vi "test_F9P.vi"() -> ()   [LabVIEW 2019] (continued)
4,3,13,13,50,315,39,14,76,037,34,28,59,310,,33,72,237,,3*7B\r\n$GBGSV,4,4,13,34,13,141,,3*47\r\n$GNGLL,3723.61643,N,12656.96813,E,064251.00,A,A*73\r\n$GNRMC,064252.00,A,3723.61654,N,12656.96823,E,0.024,,250720,,,A,V*12\r\n$GNVTG,,T,,M,0.024,N,0.044,K,A*3B\r\n$GNGGA,064252.00,3723.61654,N,12656.96823,E,1,12,0.61,43.2,M,18.5,M,,*7D\r\n$GNGSA,A,3,17,19,06,05,02,12,09,,,,,,1.08,0.61,0.89,1*0B\r\n$GNGSA,A,3,85,70,71,72,,,,,,,,,1.08,0.61,0.89,2*04\r\n$GNGSA,A,3,36,19,11,04,09,12,,,,,,,1.08,0.61,0.89,3*0F\r\n$GNGSA,A,3,28,14,13,11,33,08,10,,,,,,1.08,0.61,0.89,4*0F\r\n$GPGSV,4,1,13,02,65,334,43,04,08,037,40,05,48,261,36,06,58,076,43,1*69\r\n$GPGSV,4,2,13,07,06,105,23,09,38,057,45,12,18,263,31,13,08,191,24,1*6F\r\n$GPGSV,4,3,13,17,19,158,23,19,37,161,34,25,11,294,25,29,07,323,17,1*68\r\n$GPGSV,4,4,13,30,01,134,,1*52\r\n$GPGSV,4,1,13,02,65,334,,04,08,037,26,05,48,261,31,06,58,076,37,6*6D\r\n$GPGSV,4,2,13,07,06,105,,09,38,057,36,12,18,263,17,13,08,191,,6*6F\r\n$GPGSV,4,3,13,17,19,158,26,19,37,161,,25,11,294,,29,07,323,,6*6C\r\n$GPGSV,4,4,13,30,01,134,,6*55\r\n$GLGSV,2,1,06,70,55,030,38,71,68,223,26,72,17,216,42,84,09,133,09,1*70\r\n$GLGSV,2,2,06,85,63,111,27,86,51,337,,1*7F\r\n$GLGSV,2,1,06,70,55,030,,71,68,223,19,72,17,216,26,84,09,133,15,3*7A\r\n$GLGSV,2,2,06,85,63,111,28,86,51,337,21,3*71\r\n$GAGSV,3,1,09,02,04,287,12,04,68,085,37,09,44,196,23,11,78,037,39,7*74\r\n$GAGSV,3,2,09,12,32,115,35,18,55,284,40,19,17,042,31,25,01,241,,7*72\r\n$GAGSV,3,3,09,36,35,314,27,7*4A\r\n$GAGSV,3,1,09,02,04,287,,04,68,085,32,09,44,196,23,11,78,037,30,2*7E\r\n$GAGSV,3,2,09,12,32,115,26,18,55,284,35,19,17,042,27,25,01,241,,2*70\r\n$GAGSV,3,3,09,36,35,314,28,2*40\r\n$GBGSV,4,1,13,04,35,133,,05,09,257,,06,27,182,,07,09,201,18,1*72\r\n$GBGSV,4,2,13,08,65,355,41,09,07,194,,10,16,222,27,11,37,142,33,1*7F\r\n$GBGSV,4,3,13,13,50,315,35,14,76,037,41,28,59,310,36,33,72,237,29,1*79\r\n$GBGSV,4,4,13,34,13,141,,1*45\r\n$GBGSV,4,1,13,04,35,133,,05,09,257,,06,27,182,,07,09,201,,3*79\r\n$GBGSV,4,2,13,08,65,355,36,09,07,194,,10,16,222,18,11,37,142,32,3*70\r\n$GBGSV,4,3,13,13,50,315,39,14,76,037,33,28,59,310,,33,72,237,,3*7C\r\n$GBGSV,4,4,13,34,13,141,,3*47\r\n$GNGLL,3723.61654,N,12656.96823,E,064252.00,A,A*75\r\n$GNRMC,064253.00,A,3723.61656,N,12656.96832,E,0.099,,250720,,,A,V*17\r\n$GNVTG,,T,,M,0.099,N,0.183,K,A*37\r\n$GNGGA,064253.00,3723.61656,N,12656.96832,E,1,12,0.62,43.3,M,18.5,M,,*7C\r\n$GNGSA,A,3,17,19,06,05,02,12,09,,,,,,1.08,0.62,0.88,1*09\r\n$GNGSA,A,3,85,70,71,72,,,,,,,,,1.08,0.62,0.88,2*06\r\n$GNGSA,A,3,36,19,11,04,09,12,,,,,,,1.08,0.62,0.88,3*0D\r\n$GNGSA,A,3,28,14,13,11,33,08,10,,,,,,1.08,0.62,0.88,4*0D\r\n$GPGSV,4,1,13,02,65,334,43,04,08,037,36,05,48,261,36,06,58,076,45,1*6E\r\n$GPGSV,4,2,13,07,06,105,,09,38,057,44,12,18,263,23,13,08,191,25,1*6D\r\n$GPGSV,4,3,13,17,19,158,23,19,37,161,29,25,11,294,24,29,07,323,17,1*65\r\n$GPGSV,4,4,13,30,01,134,,1*52\r\n$GPGSV,4,1,13,02,65,334,,04,08,037,24,05,48,261,31,06,58,076,36,6*6E\r\n$GPGSV,4,2,13,07,06,105,,09,38,057,36,12,18,263,17,13,08,191,,6*6F\r\n$GPGSV,4,3,13,17,19,158,26,19,37,161,,25,11,294,,29,07,323,,6*6C\r\n$GPGSV,4,4,13,30,01,134,,6*55\r\n$GLGSV,2,1,06,70,55,030,38,71,68,223,25,72,17,216,37,84,09,133,13,1*7A\r\n$GLGSV,2,2,06,85,63,111,27,86,51,337,,1*7F\r\n$GLGSV,2,1,06,70,55,030,,71,68,223,19,72,17,216,26,84,09,133,12,3*7D\r\n$GLGSV,2,2,06,85,63,111,30,86,51,337,17,3*7D\r\n$GAGSV,3,1,09,02,04,287,09,04,68,085,39,09,44,196,30,11,78,037,38,7*73\r\n$GAGSV,3,2,09,12,32,115,30,18,55,284,33,19,17,042,31,25,01,241,,7*73\r\n$GAGSV,3,3,09,36,35,314,32,7*4E\r\n$GAGSV,3,1,09,02,04,287,,04,68,085,33,09,44,196,23,11,78,037,31,2*7E\r\n$GAGSV,3,2,09,12,32,115,26,18,55,284,35,19,17,042,26,25,01,241,,2*71\r\n$GAGSV,3,3,09,36,35,314,28,2*40\r\n$GBGSV,4,1,13,04,35,133,,05,09,257,,06,27,182,,07,09,201,20,1*79\r\n$GBGSV,4,2,13,08,65,355,39,09,07,194,,10,16,222,24,11,37,142,27,1*76\r\n$GBGSV,4,3,13,13,50,315,35,14,76,037,41,28,59,310,39,33,73,239,28,1*78\r\n$GBGSV,4,4,13,34,13,141,,1*45\r\n$GBGSV,4,1,13,04,35,133,,05,09,257,,06,27,182,,07,09,201,,3*79\r\n$GBGSV,4,2,13,08,65,355,37,09,07,194,,10,16,222,17,11,37,142,25,3*78\r\n$GBGSV,4,3,13,13,50,315,39,14,76,037,34,28,59,310,,33,73,239,,3*74\r\n$GBGSV,4,4,13,34,13,141,,3*47\r\n$GNGLL,3723.61656,N,12656.96832,E,064253.00,A,A*76\r\n$GNRMC,064254.00,A,3723.61658,N,12656.96838,E,0.064,,250720,,,A,V*16\r\n$GNVTG,,T,,M,0.064,N,0.118,K,A*37\r\n$GNGGA,064254.00,3723.61658,N,12656.96838,E,1,12,0.63,43.3,M,18.5,M,,*7E\r\n$GNGSA,A,3,17,19,06,05,02,12,09,,,,,,1.11,0.63,0.91,1*08\r\n$GNGSA,A,3,85,70,71,72,,,,,,,,,1.11,0.63,0.91,2*07\r\n$GNGSA,A,3,36,19,11,04,09,12,,,,,,,1.11,0.63,0.91,3*0C\r\n$GNGSA,A,3,28,14,13,11,33,08,10,,,,,,1.11,0.63,0.91,4*0C\r\n$GPGSV,4,1,13,02,65,334,46,04,08,037,36,05,48,261,36,06,58,076,44,1*6A\r\n$GPGSV,4,2,13,07,06,105,,09,38,057,48,12,18,263,25,13,08,191,22,1*60\r\n$GPGSV,4,3,13,17,19,158,24,19,37,161,33,25,11,294,22,29,07,323,21,1*6A\r\n$GPGSV,4,4,13,30,01,134,,1*52\r\n$GPGSV,4,1,13,02,65,334,,04,08,037,25,05,48,261,30,06,58,076,20,6*69\r\n$GPGSV,4,2,13,07,06,105,,09,38,057,38,12,18,263,16,13,08,191,,6*60\r\n$GPGSV,4,3,13,17,19,158,22,19,37,161,,25,11,294,,29,07,323,,6*68\r\n$GPGSV,4,4,13,30,01,134,,6*55\r\n$GLGSV,2,1,06,70,55,030,38,71,68,223,25,72,17,216,42,84,09,133,11,1*7A\r\n$GLGSV,2,2,06,85,63,111,34,86,51,337,,1*7D\r\n$GLGSV,2,1,06,70,55,030,,71,68,223,16,72,17,216,24,84,09,133,15,3*77\r\n$GLGSV,2,2,06,85,63,111,21,86,51,337,13,3*79\r\n$GAGSV,3,1,09,02,04,287,09,04,68,085,39,09,44,196,31,11,78,037,38,7*72\r\n$GAGSV,3,2,09,12,32,115,27,18,55,284,31,19,17,042,34,25,01,241,,7*72\r\n$GAGSV,3,3,09,36,35,314,28,7*45\r\n$GAGSV,3,1,09,02,04,287,,04,68,085,35,09,44,196,25,11,78,037,32,2*7D\r\n$GAGSV,3,2,09,12,32,115,29,18,55,284,36,19,17,042,32,25,01,241,,2*78\r\n$GAGSV,3,3,09,36,35,314,28,2*40\r\n$GBGSV,4,1,13,04,35,133,,05,09,257,,06,27,182,,07,09,201,20,1*79\r\n$GBGSV,4,2,13,08,65,355,39,09,07,194,,10,16,222,24,11,37,142,31,1*71\r\n$GBGSV,4,3,13,13,50,315,40,14,76,037,41,28,59,310,40,33,73,239,28,1*74\r\n$GBGSV,4,4,13,34,13,142,,1*46\r\n$GBGSV,4,1,13,04,35,133,,05,09,257,,06,27,182,,07,09,201,,3*79\r\n$GBGSV,4,2,13,08,65,355,37,09,07,194,,10,16,222,20,11,37,142,27,3*7E\r\n$GBGSV,4,3,13,13,50,315,40,14,76,037,34,28,59,310,,33,73,239,,3*7A\r\n$GBGSV,4,4,13,34,13,142,,3*44\r\n$GNGLL,3723.61658,N,12656.96838,E,064254.00,A,A*75\r\n$GNRMC,064255.00,A,3723.61659,N,12656.96844,E,0.055,,250720,,,A,V*1F\r\n$GNVTG,,T,,M,0.055,N,0.102,K,A*3E\r\n$GNGGA,064255.00,3723.61659,N,12656.96844,E,1,12,0.63,43.3,M,18.5,M,,*75\r\n$GNGSA,A,3,17,19,06,05,02,12,09,,,,,,1.10,0.63,0.91,1*09\r\n$GNGSA,A,3,85,70,71,72,,,,,,,,,1.10,0.63,0.91,2*06\r\n$GNGSA,A,3,36,19,11,04,09,12,,,,,,,1.10,0.63,0.91,3*0D\r\n$GNGSA,A,3,28,14,13,11,33,08,10,,,,,,1.10,0.63,0.91,4*0D\r\n$GPGSV,4,1,13,02,65,334,46,04,08,037,36,05,48,261,34,06,58,076,44,1*68\r\n$GPGSV,4,2,13,07,06,105,,09,38,057,47,12,18,263,27,13,08,191,22,1*6D\r\n$GPGSV,4,3,13,17,19,158,23,19,37,161,32,25,11,294,20,29,07,323,22,1*6D\r\n$GPGSV,4,4,13,30,01,134,,1*52\r\n$GPGSV,4,1,13,02,65,334,,04,08,037,24,05,48,261,30,06,58,076,21,6*69\r\n$GPGSV,4,2,13,07,06,105,,09,38,057,40,12,18,263,13,13,08,191,,6*6A\r\n$GPGSV,4,3,13,17,19,158,19,19,37,161,,25,11,294,,29,07,323,,6*60\r\n$GPGSV,4,4,13,30,01,134,,6*55\r\n$GLGSV,2,1,06,70,55,030,37,71,68,223,34,72,17,216,39,84,09,133,09,1*70\r\n$GLGSV,2,2,06,85,63,111,40,86,51,337,,1*7E\r\n$GLGSV,2,1,06,70,55,030,,71,68,223,16,72,17,216,26,84,09,133,17,3*77\r\n$GLGSV,2,2,06,85,63,111,29,86,51,337,13,3*71\r\n$GAGSV,3,1,09,02,04,287,09,04,68,085,41,09,44,196,30,11,78,037,39,7*7D\r\n$GAGSV,3,2,09,12,32,115,28,18,55,284,37,19,17,042,36,25,01,241,,7*79\r\n$GAGSV,3,3,09,36,35,314,33,7*4F\r\n$GAGSV,3,1,09,02,04,287,,04,68,085,35,09,44,196,25,11,78,037,33,2*7C\r\n$GAGSV,3,2,09,12,32,115,27,18,55,284,36,19,17,042,31,25,01,241,,2*75\r\n$GAGSV,3,3,09,36,35,314,27,2*4F\r\n$GBGSV,4,1,13,04,35,133,,05,09,257,,06,27,182,,07,09,201,19,1*73\r\n$GBGSV,4,2,13,08,65,355,40,09,07,194,,10,16,222,24,11,37,142,25,1*7A\r\n$GBGSV,4,3,13,13,50,315,40,14,76,037,41,28,59,310,39,33,73,239,29,1*7B\r\n$GBGSV,4,4,13,34,13,142,,1*46\r\n$GBGSV,4,1,13,04,35,133,,05,09,257,,06,27,182,,07,09,201,,3*79\r\n$GBGSV,4,2,13,08,65,355,36,09,07,194,,10,16,222,23,11,37,142,29,3*72\r\n$GBGSV,4,3,13,13,50,315,40,14,76,037,36,28,59,310,,33,73,239,,3*78\r\n$GBGSV,4,4,13,34,13,142,,3*44\r\n$GNGLL,3723.61659,N,12656.96844,E,064255.00,A,A*7E\r\n$GNRMC,064256.00,A,3723.61664,N,12656.96851,E,0.057,,250720,,,A,V*14\r\n$GNVTG,,T,,M,0.057,N,0.106,K,A*38\r\n$GNGGA,064256.00,3723.61664,N,12656.96851,E,1,12,0.61,43.5,M,18.5,M,,*78\r\n$GNGSA,A,3,17,19,06,05,02,12,09,,,,,,1.06,0.61,0.88,1*04\r\n$GNGSA,A,3,85,70,71,72,,,,,,,,,1.06,0.61,0.88,2*0B\r\n$GNGSA,A,3,36,19,11,04,09,12,,,,,,,1.06,0.61,0.88,3*00\r\n$GNGSA,A,3,28,14,13,11,33,08,10,,,,,,1.06,0.61,0.88,4*00\r\n$GPGSV,4,1,13,02,65,334,46,04,08,037,36,05,48,261,34,06,58,076,44,1*68\r\n$GPGSV,4,2,13,07,06,105,,09,38,057,47,12,18,263,28,13,08,191,22,1*62\r\n$GPGSV,4,3,13,17,19,158,24,19,37,161,32,25,11,294,21,29,07,323,23,1*6A\r\n$GPGSV,4,4,13,30,01,134,,1*52\r\n$GPGSV,4,1,13,02,65,334,,04,08,037,21,05,48,261,30,06,58,076,21,6*6C\r\n$GPGSV,4,2,13,07,06,105,,09,38,057,39,12,18,263,10,13,08,191,,6*67\r\n$GPGSV,4,3,13,17,19,158,12,19,37,161,,25,11,294,,29,07,323,,6*6B\r\n$GPGSV,4,4,13,30,01,134,,6*55\r\n$GLGSV,2,1,06,70,55,030,37,71,68,223,32,72,17,216,40,84,09,133,11,1*71\r\n$GLGSV,2,2,06,85,63,111,39,86,51,337,,1*70\r\n$GLGSV,2,1,06,70,55,030,,71,68,223,16,72,17,216,27,84,09,133,17,3*76\r\n$GLGSV,2,2,06,85,63,111,28,86,51,337,16,3*75\r\n$GAGSV,3,1,09,02,04,287,09,04,68,085,42,09,44,196,29,11,78,037,39,7*76\r\n$GAGSV,3,2,09,12,32,115,29,18,55,284,37,19,17,042,34,25,01,241,,7*7A\r\n$GAGSV,3,3,09,36,35,314,32,7*4E\r\n$GAGSV,3,1,09,02,04,287,,04,68,085,36,09,44,196,25,11,78,037,33,2*7F\r\n$GAGSV,3,2,09,12,32,115,27,18,55,284,36,19,17,042,30,25,01,241,,2*74\r\n$GAGSV,3,3,09,36,35,314,27,2*4F\r\n$GBGSV,4,1,13,04,35,133,,05,09,257,,06,27,182,,07,09,201,17,1*7D\r\n$GBGSV,4,2,13,08,65,355,40,09,07,194,,10,16,222,23,11,37,142,27,1*7F\r\n$GBGSV,4,3,13,13,50,315,40,14,76,037,41,28,59,310,39,33,73,239,29,1*7B\r\n$GBGSV,4,4,13,34,13,142,,1*46\r\n$GBGSV,4,1,13,04,35,133,,05,09,257,,06,27,182,,07,09,201,,3*79\r\n$GBGSV,4,2,13,08,65,355,37,09,07,194,,10,16,222,25,11,37,142,30,3*7D\r\n$GBGSV,4,3,13,13,50,315,40,14,76,037,36,28,59,310,,33,73,239,,3*78\r\n$GBGSV,4,4,13,34,13,142,,3*44\r\n$GNGLL,3723.61664,N,12656.96851,E,064256.00,A,A*77\r\n$GNRMC,064257.00,A,3723.61665,N,12656.96856,E,0.034,,250720,,,A,V*16\r\n$GNVTG,,T,,M,0.034,N,0.063,K,A*3F\r\n$GNGGA,064257.00,3723.61665,N,12656.96856,E,1,12,0.62,43.6,M,18.5,M,,*7F\r\n$GNGSA,A,3,17,19,06,05,02,12,09,,,,,,1.10,0.62,0.90,1*09\r\n$GNGSA,A,3,85,70,71,72,,,,,,,,,1.10,0.62,0.90,2*06\r\n$GNGSA,A,3,36,19,11,04,09,12,,,,,,,1.10,0.62,0.90,3*0D\r\n$GNGSA,A,3,28,14,13,11,33,08,10,,,,,,1.10,0.62,0.90,4*0D\r\n$GPGSV,4,1,13,02,65,334,46,04,08,037,35,05,48,261,35,06,58,076,44,1*6A\r\n$GPGSV,4,2,13,07,06,105,,09,38,057,48,12,18,263,27,13,08,191,23,1*63\r\n$GPGSV,4,3,13,17,19,158,26,19,37,161,31,25,11,294,,29,07,323,23,1*68\r\n$GPGSV,4,4,13,30,01,134,,1*52\r\n$GPGSV,4,1,13,02,65,334,,04,08,037,18,05,48,261,29,06,58,076,20,6*6F\r\n$GPGSV,4,2,13,07,06,105,,09,38,057,40,12,18,263,,13,08,191,,6*68\r\n$GPGSV,4,3,13,17,19,158,12,19,37,161,,25,11,294,,29,07,323,,6*6B\r\n$GPGSV,4,4,13,30,01,134,,6*55\r\n$GLGSV,2,1,06,70,55,030,38,71,68,223,32,72,17,216,40,84,09,133,12,1*7D\r\n$GLGSV,2,2,06,85,63,111,39,86,51,337,,1*70\r\n$GLGSV,2,1,06,70,55,030,,71,68,223,17,72,17,216,27,84,09,133,17,3*77\r\n$GLGSV,2,2,06,85,63,111,28,86,51,337,17,3*74\r\n$GAGSV,3,1,09,02,04,287,13,04,68,085,42,09,44,196,29,11,78,037,39,7*7D\r\n$GAGSV,3,2,09,12,32,115,29,18,55,284,37,19,17,042,34,25,01,241,,7*7A\r\n$GAGSV,3,3,09,36,35,314,32,7*4E\r\n$GAGSV,3,1,09,02,04,287,,04,68,085,36,09,44,196,25,11,78,037,33,2*7F\r\n$GAGSV,3,2,09,12,32,115,26,18,55,284,36,19,17,042,30,25,01,241,,2*75\r\n$GAGSV,3,3,09,36,35,314,27,2*4F\r\n$GBGSV,4,1,13,04,35,133,,05,09,257,,06,27,182,,07,09,201,,1*7B\r\n$GBGSV,4,2,13,08,65,355,40,09,07,194,,10,16,222,23,11,37,142,27,1*7F\r\n$GBGSV,4,3,13,13,50,315,40,14,76,037,42,28,59,310,39,33,73,239,28,1*79\r\n$GBGSV,4,4,13,34,13,142,,1*46\r\n$GBGSV,4,1,13,04,35,133,,05,09,257,,06,27,182,,07,09,201,,3*79\r\n$GBGSV,4,2,13,08,65,355,37,09,07,194,,10,16,222,25,11,37,142,32,3*7F\r\n$GBGSV,4,3,13,13,50,315,40,14,76,037,36,28,59,310,,33,73,239,,3*78\r\n$GBGSV,4,4,13,34,13,142,,3*44\r\n$GNGLL,3723.61665,N,12656.96856,E,064257.00,A,A*70\r\n$GNRMC,064258.00,A,3723.61669,N,12656.96861,E,0.056,,250720,,,A,V*15\r\n$GNVTG,,T,,M,0.056,N,0.103,K,A*3C\r\n$GNGGA,064258.00,3723.61669,N,12656.96861,E,1,12,0.62,43.7,M,18.5,M,,*79\r\n$GNGSA,A,3,17,19,06,05,02,12,09,,,,,,1.10,0.62,0.90,1*09\r\n$GNGSA,A,3,85,70,71,72,,,,,,,,,1.10,0.62,0.90,2*06\r\n$GNGSA,A,3,36,19,11,04,09,12,,,,,,,1.10,0.62,0.90,3*0D\r\n$GNGSA,A,3,28,14,13,11,33,08,10,,,,,,1.10,0.62,0.90,4*0D\r\n$GPGSV,4,1,13,02,65,334,46,04,08,037,35,05,48,261,35,06,58,076,44,1*6A\r\n$GPGSV,4,2,13,07,06,105,,09,38,057,48,12,18,263,25,13,08,191,22,1*60\r\n$GPGSV,4,3,13,17,19,158,27,19,37,161,32,25,11,294,,29,07,323,23,1*6A\r\n$GPGSV,4,4,13,30,01,134,,1*52\r\n$GPGSV,4,1,13,02,65,334,,04,08,037,19,05,48,261,30,06,58,076,20,6*66\r\n$GPGSV,4,2,13,07,06,105,,09,38,057,43,12,18,263,,13,08,191,,6*6B\r\n$GPGSV,4,3,13,17,19,158,14,19,37,161,,25,11,294,,29,07,323,,6*6D\r\n$GPGSV,4,4,13,30,01,134,,6*55\r\n$GLGSV,2,1,06,70,55,030,38,71,68,223,33,72,17,216,39,84,09,133,12,1*72\r\n$GLGSV,2,2,06,85,63,111,39,86,51,337,,1*70\r\n$GLGSV,2,1,06,70,55,030,,71,68,223,18,72,17,216,26,84,09,133,16,3*78\r\n$GLGSV,2,2,06,85,63,111,28,86,51,337,18,3*7B\r\n$GAGSV,3,1,09,02,04,287,11,04,68,085,41,09,44,196,30,11,78,037,39,7*74\r\n$GAGSV,3,2,09,12,32,115,28,18,55,284,37,19,17,042,34,25,01,241,,7*7B\r\n$GAGSV,3,3,09,36,35,314,32,7*4E\r\n$GAGSV,3,1,09,02,04,287,,04,68,085,35,09,44,196,25,11,78,037,35,2*7A\r\n$GAGSV,3,2,09,12,32,115,24,18,55,284,37,19,17,042,30,25,01,241,,2*76\r\n$GAGSV,3,3,09,36,35,314,26,2*4E\r\n$GBGSV,4,1,13,04,35,133,,05,09,257,,06,27,182,,07,09,201,,1*7B\r\n$GBGSV,4,2,13,08,65,355,39,09,07,194,,10,16,222,22,11,37,142,27,1*70\r\n$GBGSV,4,3,13,13,50,315,40,14,76,037,42,28,59,310,39,33,73,239,28,1*79\r\n$GBGSV,4,4,13,34,13,142,,1*46\r\n$GBGSV,4,1,13,04,35,133,,05,09,257,,06,27,182,,07,09,201,,3*79\r\n$GBGSV,4,2,13,08,65,355,39,09,07,194,,10,16,222,26,11,37,142,35,3*75\r\n$GBGSV,4,3,13,13,50,315,43,14,76,037,38,28,59,310,,33,73,239,,3*75\r\n$GBGSV,4,4,13,34,13,142,,3*44\r\n$GNGLL,3723.61669,N,12656.96861,E,064258.00,A,A*77\r\n$GNRMC,064259.00,A,3723.61674,N,12656.96865,E,0.025,,250720,,,A,V*18\r\n$GNVTG,,T,,M,0.025,N,0.047,K,A*39\r\n$GNGGA,064259.00,3723.61674,N,12656.96865,E,1,12,0.63,43.8,M,18.5,M,,*7E\r\n$GNGSA,A,3,17,19,06,05,02,12,09,,,,,,1.10,0.63,0.91,1*09\r\n$GNGSA,A,3,85,70,71,72,,,,,,,,,1.10,0.63,0.91,2*06\r\n$GNGSA,A,3,36,19,11,04,09,12,,,,,,,1.10,0.63,0.91,3*0D\r\n$GNGSA,A,3,28,14,13,11,33,08,10,,,,,,1.10,0.63,0.91,4*0D\r\n$GPGSV,4,1,13,02,65,334,45,04,08,037,36,05,48,261,36,06,58,076,44,1*69\r\n$GPGSV,4,2,13,07,06,105,,09,38,057,49,12,18,263,24,13,08,191,22,1*60\r\n$GPGSV,4,3,13,17,19,158,28,19,37,161,31,25,11,294,,29,07,323,22,1*67\r\n$GPGSV,4,4,13,30,01,134,,1*52\r\n$GPGSV,4,1,13,02,65,334,,04,08,037,21,05,48,261,31,06,58,076,17,6*68\r\n$GPGSV,4,2,13,07,06,105,20,09,38,057,41,12,18,263,,13,08,191,20,6*69\r\n$GPGSV,4,3,13,17,19,158,15,19,37,161,,25,11,294,,29,07,323,,6*6C\r\n$GPGSV,4,4,13,30,01,134,,6*55\r\n$GLGSV,2,1,06,70,55,030,39,71,68,223,34,72,17,216,38,84,09,133,08,1*7E\r\n$GLGSV,2,2,06,85,63,111,39,86,51,337,,1*70\r\n$GLGSV,2,1,06,70,55,030,,71,68,223,20,72,17,216,26,84,09,133,18,3*7D\r\n$GLGSV,2,2,06,85,63,111,28,86,51,337,19,3*7A\r\n$GAGSV,3,1,09,02,04,287,08,04,68,085,42,09,44,196,30,11,78,037,39,7*7F\r\n$GAGSV,3,2,09,12,32,115,27,18,55,284,37,19,17,042,34,25,01,241,,7*74\r\n$GAGSV,3,3,09,36,35,314,32,7*4E\r\n$GAGSV,3,1,09,02,04,287,,04,68,085,35,09,44,196,26,11,78,037,34,2*78\r\n$GAGSV,3,2,09,12,32,115,24,18,55,284,37,19,17,042,31,25,01,241,,2*77\r\n$GAGSV,3,3,09,36,35,314,26,2*4E\r\n$GBGSV,4,1,13,04,35,133,,05,09,257,,06,27,182,,07,09,201,,1*7B\r\n$GBGSV,4,2,13,08,65,355,39,09,07,194,,10,16,222,22,11,37,142,27,1*70\r\n$GBGSV,4,3,13,13,50,315,40,14,76,037,42,28,59,310,39,33,73,239,29,1*78\r\n$GBGSV,4,4,13,34,13,142,,1*46\r\n$GBGSV,4,1,13,04,35,133,,05,09,257,,06,27,182,,07,09,201,,3*79\r\n$GBGSV,4,2,13,08,65,355,38,09,07,194,,10,16,222,25,11,37,142,34,3*76\r\n$GBGSV,4,3,13,13,50,315,42,14,76,037,37,28,59,310,,33,73,239,,3*7B\r\n$GBGSV,4,4,13,34,13,142,,3*44\r\n$GNGLL,3723.61674,N,12656.96865,E,064259.00,A,A*7E\r\n$GNRMC,064300.00,A,3723.61677,N,12656.96870,E,0.009,,250720,,,A,V*1C\r\n$GNVTG,,T,,M,0.009,N,0.016,K,A*33\r\n$GNGGA,064300.00,3723.61677,N,12656.96870,E,1,12,0.63,43.8,M,18.5,M,,*74\r\n$GNGSA,A,3,17,19,06,05,02,12,09,,,,,,1.10,0.63,0.91,1*09\r\n$GNGSA,A,3,85,70,71,72,,,,,,,,,1.10,0.63,0.91,2*06\r\n$GNGSA,A,3,36,19,11,04,09,12,,,,,,,1.10,0.63,0.91,3*0D\r\n$GNGSA,A,3,28,14,13,11,33,08,10,,,,,,1.10,0.63,0.91,4*0D\r\n$GPGSV,4,1,13,02,65,334,45,04,08,037,35,05,48,261,35,06,58,076,45,1*68\r\n$GPGSV,4,2,13,07,06,105,,09,38,057,49,12,18,263,23,13,08,191,21,1*64\r\n$GPGSV,4,3,13,17,19,158,27,19,37,161,29,25,11,294,,29,07,323,22,1*61\r\n$GPGSV,4,4,13,30,01,134,,1*52\r\n$GPGSV,4,1,13,02,65,334,,04,08,037,23,05,48,261,31,06,58,076,17,6*6A\r\n$GPGSV,4,2,13,07,06,105,17,09,38,057,40,12,18,263,18,13,08,191,16,6*60\r\n$GPGSV,4,3,13,17,19,158,16,19,37,161,,25,11,294,,29,07,323,,6*6F\r\n$GPGSV,4,4,13,30,01,134,,6*55\r\n$GLGSV,2,1,06,70,55,030,39,71,68,223,34,72,17,216,38,84,09,133,10,1*77\r\n$GLGSV,2,2,06,85,63,111,38,86,51,337,,1*71\r\n$GLGSV,2,1,06,70,55,030,,71,68,223,21,72,17,216,25,84,09,133,18,3*7F\r\n$GLGSV,2,2,06,85,63,111,29,86,51,337,20,3*71\r\n$GAGSV,3,1,09,02,04,287,10,04,68,085,42,09,44,196,31,11,78,037,39,7*77\r\n$GAGSV,3,2,09,12,32,115,28,18,55,284,37,19,17,042,34,25,01,241,,7*7B\r\n$GAGSV,3,3,09,36,35,314,32,7*4E\r\n$GAGSV,3,1,09,02,04,287,,04,68,085,36,09,44,196,27,11,78,037,34,2*7A\r\n$GAGSV,3,2,09,12,32,115,24,18,55,284,37,19,17,042,31,25,01,241,,2*77\r\n$GAGSV,3,3,09,36,35,314,26,2*4E\r\n$GBGSV,4,1,13,04,35,133,,05,09,257,,06,27,182,,07,09,201,,1*7B\r\n$GBGSV,4,2,13,08,65,355,39,09,07,194,,10,16,222,22,11,37,142,25,1*72\r\n$GBGSV,4,3,13,13,50,315,40,14,76,037,42,28,59,310,38,33,73,239,29,1*79\r\n$GBGSV,4,4,13,34,13,142,,1*46\r\n$GBGSV,4,1,13,04,35,133,,05,09,257,,06,27,182,,07,09,201,,3*79\r\n$GBGSV,4,2,13,08,65,355,38,09,07,194,,10,16,222,26,11,37,142,34,3*75\r\n$GBGSV,4,3,13,13,50,315,42,14,76,037,37,28,59,310,,33,73,239,,3*7B\r\n$GBGSV,4,4,13,34,13,142,,3*44\r\n$GNGLL,3723.61677,N,12656.96870,E,064300.00,A,A*74\r\n$GNRMC,064301.00,A,3723.61677,N,12656.96875,E,0.040,,250720,,,A,V*15\r\n$GNVTG,,T,,M,0.040,N,0.074,K,A*3A\r\n$GNGGA,064301.00,3723.61677,N,12656.96875,E,1,12,0.63,43.9,M,18.5,M,,*71\r\n$GNGSA,A,3,17,19,06,05,02,12,09,,,,,,1.10,0.63,0.91,1*09\r\n$GNGSA,A,3,85,70,71,72,,,,,,,,,1.10,0.63,0.91,2*06\r\n$GNGSA,A,3,36,19,11,04,09,12,,,,,,,1.10,0.63,0.91,3*0D\r\n$GNGSA,A,3,28,14,13,11,33,08,10,,,,,,1.10,0.63,0.91,4*0D\r\n$GPGSV,4,1,13,02,65,334,45,04,08,037,35,05,48,261,35,06,58,076,45,1*68\r\n$GPGSV,4,2,13,07,06,105,,09,38,057,48,12,18,263,22,13,08,191,21,1*64\r\n$GPGSV,4,3,13,17,19,158,26,19,37,161,29,25,11,294,,29,07,323,22,1*60\r\n$GPGSV,4,4,13,30,01,134,,1*52\r\n$GPGSV,4,1,13,02,65,334,,04,08,037,22,05,48,261,32,06,58,076,21,6*6D\r\n$GPGSV,4,2,13,07,06,105,11,09,38,057,41,12,18,263,15,13,08,191,,6*6D\r\n$GPGSV,4,3,13,17,19,158,17,19,37,161,,25,11,294,,29,07,323,,6*6E\r\n$GPGSV,4,4,13,30,01,134,,6*55\r\n$GLGSV,2,1,06,70,55,030,36,71,68,223,36,72,17,216,37,84,09,133,09,1*7D\r\n$GLGSV,2,2,06,85,63,111,40,86,51,337,,1*7E\r\n$GLGSV,2,1,06,70,55,030,,71,68,223,21,72,17,216,23,84,09,133,12,3*73\r\n$GLGSV,2,2,06,85,63,111,28,86,51,337,19,3*7A\r\n$GAGSV,3,1,09,02,04,287,10,04,68,085,42,09,44,196,31,11,78,037,39,7*77\r\n$GAGSV,3,2,09,12,32,115,28,18,55,284,37,19,17,042,34,25,01,241,,7*7B\r\n$GAGSV,3,3,09,36,35,314,32,7*4E\r\n$GAGSV,3,1,09,02,04,287,,04,68,
